vi "avec choix du calcul.vi"() -> ()   [LabVIEW 2014]
panel:
  out "resultat":dbl
  in  "number  2":dbl
  in  "number 1":dbl
  in  "operation":u16(ring) items=["+", "sous", "*", "/", "moy"]
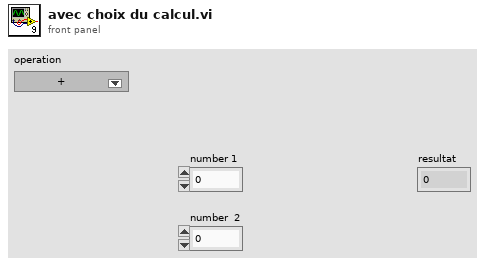
[diagram p1: front panel]
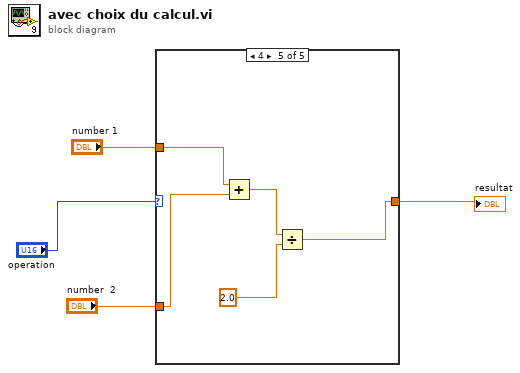
[diagram p0: block diagram]
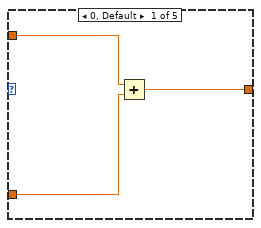
[diagram p2: hidden frame]
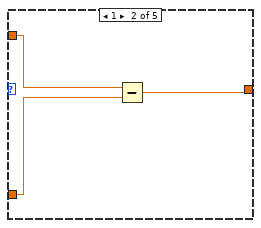
[diagram p3: hidden frame]
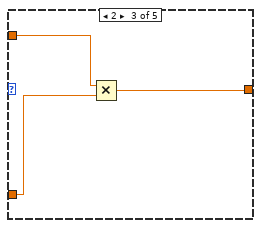
[diagram p4: hidden frame]
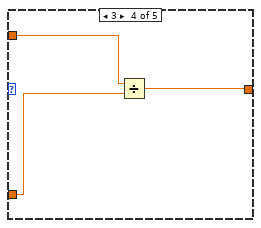
[diagram p5: hidden frame]
diagram:
  n1 = case shown="4" "operation" {
    tunnel: "number 1" -> [w7 w10 w13 w16 w18]
    tunnel: "number  2" -> [w6 w9 w12 w15 w17]
    tunnel: [w5 w8 w11 w14 w19] -> w1
    frame 0, Default {
      n2 = Add(x=w7, y=w6) -> (x+y=w5:dbl)
    }
    frame 1 {
      n3 = Subtract(x=w10, y=w9) -> (x-y=w8:dbl)
    }
    frame 2 {
      n4 = Multiply(x=w13, y=w12) -> (x*y=w11:dbl)
    }
    frame 3 {
      n5 = Divide(x=w16, y=w15) -> (x/y=w14:dbl)
    }
    frame 4 {
      n6 = Add(x=w18, y=w17) -> (x+y=w20:dbl)
      n7 = Divide(x=w20, y=2.0) -> (x/y=w19:dbl)
    }
  }
  "resultat" <- w1
